vi "Dereference Bitmap Glyph.vi"(8 "error in (no error)":errorcluster, 11 "glyph ref in":i64) -> (0 "error out":errorcluster, 2 "Bitmap Glyph Rec":T1, 3 "glyph ref out":i64)   [LabVIEW 2023, in "Freetype Drawer.lvlib"]
uses:
  Freetype Drawer.lvlib
  Bitmap Glyph.ctl
  Glyph Rec.ctl
  FT Bitmap.ctl
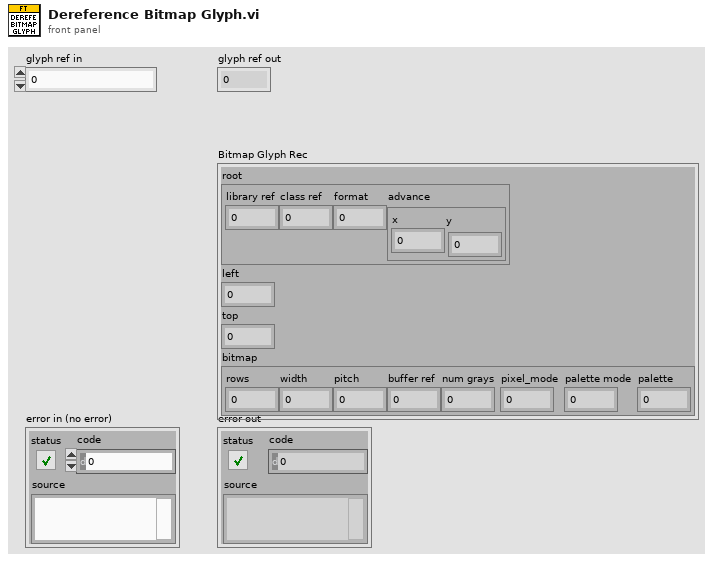
[diagram p1: front panel]
types:
  T1 = typedef "Freetype Drawer.lvlib/Bitmap Glyph.ctl" = cluster{"root":T2, "left":i32, "top":i32, "bitmap":T3}
  T2 = typedef "Freetype Drawer.lvlib/Glyph Rec.ctl" = cluster{"library ref":i64, "class ref":i64, "format":i32, "advance":cluster{"x":i32, "y":i32}}
  T3 = typedef "Freetype Drawer.lvlib/FT Bitmap.ctl" = cluster{"rows":u32, "width":u32, "pitch":i32, "buffer ref":i64, "num grays":i16, "pixel_mode":u8, "palette mode":u8, "palette":i64}
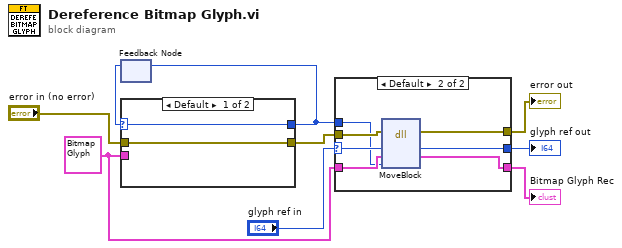
[diagram p0: block diagram]
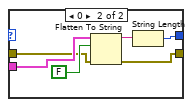
[diagram p3: hidden frame]
diagram:
  w8 = T1 {"root"={"library ref"=0, "class ref"=0, "format"=0, "advance"={"x"=0, "y"=0}}, "left"=0, "top"=0, "bitmap"={"rows"=0, "width"=0, "pitch"=0, "buffer ref"=0, "num grays"=0, "pixel_mode"=0, "palette mode"=0, "palette"=0}} ("Bitmap Glyph")
  n1 = feedback #1() -> (w1:i32)  [unwired: 1 in]
  n2 = case shown="Default" w1 {
    selector: w1 -> [w11 _]
    tunnel: w8 -> [_ w15]
    tunnel: "error in (no error)" -> [w10 w14]
    tunnel: [w10 w13] -> w4
    tunnel: [w11 w12] -> w2
    frame Default {
    }
    frame 0 {
      n3 = Flatten To String(anything=w15, prepend array or string size? (T)=FALSE, error in (no error)=w14) -> (data string=w17:string, error out=w13:errorcluster)  [unwired: 1 in, 1 out]
      n4 = String Length(string=w17) -> (length=w12:i32)
    }
  }
  n5 = feedback-in #1(w2) -> ()
  n6 = case shown="Default" "glyph ref in" {
    selector: "glyph ref in" -> [w20 w24]
    tunnel: [w19 w27] -> w9
    tunnel: w8 -> [w18 w26]
    tunnel: [w20 w25] -> w7
    tunnel: w4 -> [w19 w23]
    tunnel: [w18 w22] -> w3
    tunnel: w2 -> [_ w21]
    frame 0 {
    }
    frame Default {
      n7 = dll-call lib="LabVIEW" fn="MoveBlock"(error in=w23, "in"=w24, "out"=w26, "size"=w21) -> (error out=w27:errorcluster, "in"=w25:i64, "out"=w22:T1)  [unwired: 4 in, 1 out]
    }
  }
  "error out" <- w9
  "glyph ref out" <- w7
  "Bitmap Glyph Rec" <- w3
